vi "Model Initial Values - Please Wait Dialog.vi"(1 "notifier out":refnum<notifier>) -> (0 "Boolean":bool)   [LabVIEW 2011, in "Model Initial Values Custom Device.lvlib"]
uses:
  Model Initial Values Custom Device.lvlib
panel:
  # "Please Wait While The Operation Completes..."
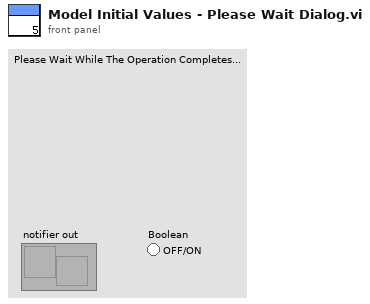
[diagram p1: front panel]
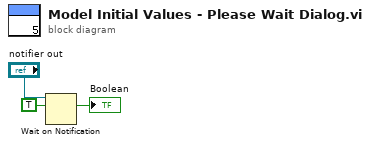
[diagram p0: block diagram]
diagram:
  n1 = Wait on Notification(notifier="notifier out", ignore previous (F)=TRUE) -> (notification=→"Boolean":bool)  [unwired: 2 in, 3 out]
